vi "5668 Configure Scan with External LO.vi"(0 "IVI Refnum in":refnum<k15>="RFSA" caption="Resource Name RFSA", 1 "Resource Name RFSG LO Generation":refnum<k15>="RFSG" caption="resource name", 2 "Start Carrier Frequency (Hz)":dbl format="%#_6p", 3 "Stop Carrier Frequency (Hz)":dbl=6000000000.0 format="%#_6p", 4 "Reference Level (dBm)":dbl format="%.2f", 5 "error in":errorcluster, 6 "source":T1="PXI_Trig0" caption="Trigger Source", 7 "output terminal":T2="PXI_Trig1", 9 "Resolution Bandwidth (Hz)":dbl=10000.0 format="%#_6p") -> (14 "RFSA Instrument Handle Out":refnum<k15>, 15 "RFSG instrument handle out":refnum<k15>, 19 "error out":errorcluster)   [LabVIEW 2017]
uses:
  <instrlib>/niRFSA/niRFSA.llb/niRFSA Exported Signal Destinations.ctl
  <instrlib>/niRFSA/niRFSA.llb/niRFSA Trigger Terminals.ctl
  <instrlib>/niRFSA/niRFSA.llb/niRFSA Acquisition Types.ctl
  <instrlib>/niRFSA/niRFSA.llb/niRFSA Signal Names.ctl
  <instrlib>/niRFSA/niRFSA.llb/niRFSA Ref Clock Sources.ctl
  <instrlib>/niRFSA/niRFSA.llb/niRFSA Configure Digital Edge Advance Trigger.vi
  <instrlib>/niRFSA/niRFSA.llb/niRFSA Configure Digital Edge Start Trigger.vi
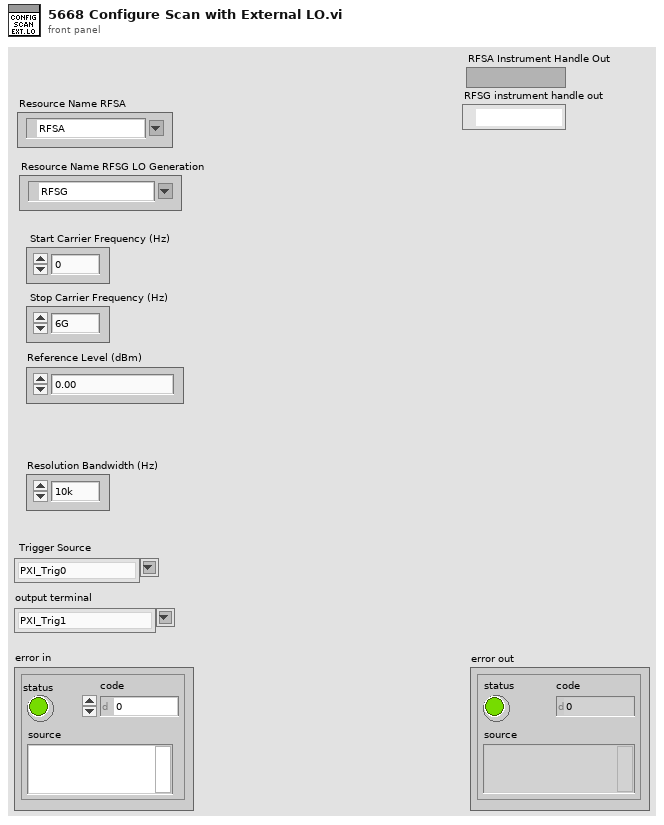
[diagram p1: front panel]
types:
  T1 = typedef "niRFSA Trigger Terminals.ctl" = string
  T2 = typedef "niRFSA Exported Signal Destinations.ctl" = string
  T3 = typedef "niRFSA Ref Clock Sources.ctl" = string
  T4 = typedef "niRFSA Signal Names.ctl" = i32
  T5 = typedef "niRFSA Acquisition Types.ctl" = i32
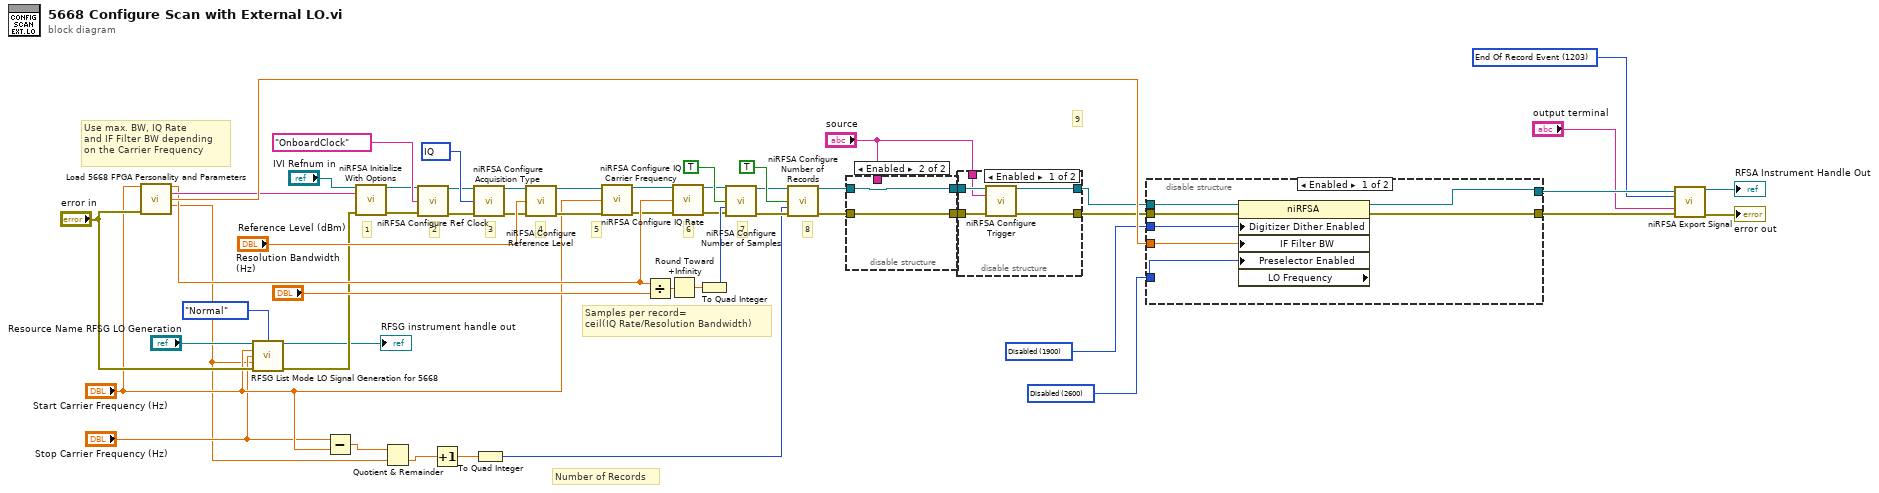
[diagram p0: block diagram]
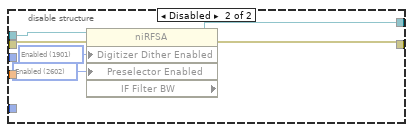
[diagram p2: hidden frame]
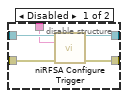
[diagram p4: hidden frame]
diagram:
  w51 = 2600 items=["Disabled"=2600, "Enabled when in Signal Path"=2601, "Enabled"=2602] ("Signal Path:Advanced:Downconverter Preselector Enabled")
  w50 = 1900 items=["Disabled"=1900, "Enabled"=1901] ("Signal Path:Digitizer Dither Enabled")
  w30 = T4 1203 items=["Start Trigger"=1100, "Ref Trigger"=702, "Advance Trigger"=1102, "Ready For Start Event"=1200, "Ready For Ref Event"=1201, "Ready For Advance Event"=1202, "End Of Record Event"=1203, "Done Event"=1204, "Reference Clock"=1205, "User"=1206] ("signal")
  w27 = T5 100 items=["IQ"=100, "Spectrum"=101] ("acquisition type")
  # "Number of Records"
  # "Use max. BW, IQ Rate \nand IF Filter BW depending \non the Carrier Frequency"
  # "Samples per record= \nceil(IQ Rate/Resolution Bandwidth)"
  # "9"
  # "8"
  # "7"
  # "6"
  # "5"
  # "4"
  # "3"
  # "2"
  # "1"
  n1 = call "Load 5668 FPGA Personality and Parameters.vi"("Start Carrier Frequency in"="Start Carrier Frequency (Hz)", "error in"="error in") -> ("IQ rate (S/s)"=w52:dbl, "option string"=w53:string, "Signal Path:IF Filter Bandwidth"=w54:dbl, "Spacing Center Frequencies"=w4:dbl)  [unwired: 9 in, 1 out]
  n2 = call "RFSG List Mode LO Signal Generation for 5668.vi"("Resource Name"="Resource Name RFSG LO Generation", "Mode"=enum16{"Normal", "Measure Flatness"}."Normal", "Start Frequency"="Start Carrier Frequency (Hz)", "End Frequency"="Stop Carrier Frequency (Hz)", "Spacing"=w4, "error in"="error in") -> ("instrument handle out"=→"RFSG instrument handle out":refnum<k15>, "error out"=w10:errorcluster)  [unwired: 8 in]
  n3 = Subtract(x="Stop Carrier Frequency (Hz)", y="Start Carrier Frequency (Hz)") -> (x-y=w5:dbl)
  n4 = call <instrlib>:"niRFSA Initialize With Options.vi"("resource name"="IVI Refnum in", "option string"=w53, "error in"=w10) -> ("instrument handle out"=w13:refnum<k15>, "error out"=w14:errorcluster)  [unwired: 11 in]
  n5 = Quotient & Remainder(x=w5, y=w4) -> (floor(x/y)=w1:dbl)  [unwired: 1 out]
  n6 = call <instrlib>:"niRFSA Configure Ref Clock.vi"("instrument handle"=w13, "clock source"=T3 "OnboardClock" ("Clock Source"), "error in"=w14) -> ("instrument handle out"=w18:refnum<k15>, "error out"=w17:errorcluster)  [unwired: 11 in]
  n7 = Increment(x=w1) -> (x+1=w3:dbl)
  n8 = call <instrlib>:"niRFSA Configure Acquisition Type.vi"("instrument handle"=w18, "acquisition type"=w27, "error in"=w17) -> ("instrument handle out"=w15:refnum<k15>, "error out"=w16:errorcluster)  [unwired: 11 in]
  n9 = To Quad Integer(1:w3) -> (0:w2:i64)
  n10 = call <instrlib>:"niRFSA Configure Reference Level.vi"("instrument handle"=w15, "reference level (dBm)"="Reference Level (dBm)", "error in"=w16) -> ("instrument handle out"=w34:refnum<k15>, "error out"=w36:errorcluster)  [unwired: 11 in]
  n11 = call <instrlib>:"niRFSA Configure IQ Carrier Frequency.vi"("instrument handle"=w34, "carrier frequency"="Start Carrier Frequency (Hz)", "error in"=w36) -> ("instrument handle out"=w35:refnum<k15>, "error out"=w37:errorcluster)  [unwired: 11 in]
  n12 = Divide(x=w52, y="Resolution Bandwidth (Hz)") -> (x/y=w44:dbl)
  n13 = Round Toward +Infinity(x=w44) -> (ceil(x): smallest int >= x=w45:dbl)
  n14 = call <instrlib>:"niRFSA Configure IQ Rate.vi"("instrument handle"=w35, "IQ rate (S/s)"=w52, "error in"=w37) -> ("instrument handle out"=w20:refnum<k15>, "error out"=w19:errorcluster)  [unwired: 11 in]
  n15 = To Quad Integer(1:w45) -> (0:w46:i64)
  n16 = call <instrlib>:"niRFSA Configure Number of Samples.vi"("instrument handle"=w20, "number of samples is finite"=TRUE, "samples per record"=w46, "error in"=w19) -> ("instrument handle out"=w23:refnum<k15>, "error out"=w24:errorcluster)  [unwired: 10 in]
  n17 = call <instrlib>:"niRFSA Configure Number of Records.vi"("instrument handle"=w23, "number of records is finite"=TRUE, "number of records"=w2, "error in"=w24) -> ("instrument handle out"=w40:refnum<k15>, "error out"=w29:errorcluster)  [unwired: 10 in]
  n18 = disable-structure shown="Enabled" {
    disable-tunnel: w29 -> [w59 w60]
    disable-tunnel: [w58 w60] -> w39
    disable-tunnel: w40 -> [w57 w61]
    disable-tunnel: [w56 w61] -> w41
    disable-tunnel: "source" -> [w55 _]
    frame Disabled {
      n19 = call-poly <instrlib>:"niRFSA Configure Trigger.vi"("instrument handle"=w57, "source"=w55, "error in"=w59) -> ("instrument handle out"=w56:refnum<k15>, "error out"=w58:errorcluster)  [unwired: 11 in]
    }
    frame Enabled {
    }
  }
  n20 = disable-structure shown="Enabled" {
    disable-tunnel: [w66 w67] -> w38
    disable-tunnel: [w65 w68] -> w48
    disable-tunnel: w39 -> [w64 w67]
    disable-tunnel: w41 -> [w63 w68]
    disable-tunnel: "source" -> [w62 _]
    frame Enabled {
      n21 = call-poly <instrlib>:"niRFSA Configure Trigger.vi"("instrument handle"=w63, "source"=w62, "error in"=w64) -> ("instrument handle out"=w65:refnum<k15>, "error out"=w66:errorcluster)  [unwired: 11 in]
    }
    frame Disabled {
    }
  }
  n22 = disable-structure shown="Enabled" {
    disable-tunnel: w38 -> [w75 w80]
    disable-tunnel: [w74 w79] -> w47
    disable-tunnel: w48 -> [w73 w82]
    disable-tunnel: [w72 w81] -> w49
    disable-tunnel: w50 -> [w71 _]
    disable-tunnel: w51 -> [w70 _]
    disable-tunnel: w54 -> [w69 _]
    frame Enabled {
      n23 = property class="niRFSA" props=["Digitizer Dither Enabled", "IF Filter BW", "Preselector Enabled", "LO Frequency"](reference=w73, error in=w75, "Digitizer Dither Enabled"=w71, "IF Filter BW"=w69, "Preselector Enabled"=w70) -> (reference out=w72:refnum<k15>, error out=w74:errorcluster)  [unwired: 1 out]
    }
    frame Disabled {
      w77 = 2602 items=["Disabled"=2600, "Enabled when in Signal Path"=2601, "Enabled"=2602] ("Signal Path:Advanced:Downconverter Preselector Enabled")
      w78 = 1901 items=["Disabled"=1900, "Enabled"=1901] ("Signal Path:Digitizer Dither Enabled")
      n24 = property class="niRFSA"(reference=w82, error in=w80, "Digitizer Dither Enabled"=w78, "Preselector Enabled"=w77) -> (reference out=w81:refnum<k15>, error out=w79:errorcluster, "IF Filter BW"=w76:dbl)
    }
  }
  n25 = call <instrlib>:"niRFSA Export Signal.vi"("instrument handle"=w49, "signal"=w30, "output terminal"="output terminal", "error in"=w47) -> ("instrument handle out"=→"RFSA Instrument Handle Out":refnum<k15>, "error out"=→"error out":errorcluster)  [unwired: 10 in]
